vi "Configure Sweep Mode.vi"(5 "Return Time (1s)":dbl[unit]=1.0 format="%#.6g", 7 "Hold Time (0 s)":dbl[unit] format="%#.6g", 8 "error in (no error)":errorcluster, 9 "Sweep Mode (0: Repeated)":u16(ring) items=["Repeated", "Triggered"], 10 "Channel  (0: Channel 1)":T1 items=["Channel 1", "Channel 2"], 11 "VISA resource name":refnum<visa-resource-name>) -> (0 "error out":errorcluster, 3 "VISA resource name out":refnum<visa-resource-name>)   [LabVIEW 2009, in "Tektronix AFG 3000 Series.lvlib"]
doc: "Configures the sweep mode. The VI decides whether the function generator produces a sweep when it receives a trigger or continuous sweep at a rate spedified by sweep time, hold time and return time."
uses:
  Tektronix AFG 3000 Series.lvlib
  controls.llb/Channel.ctl
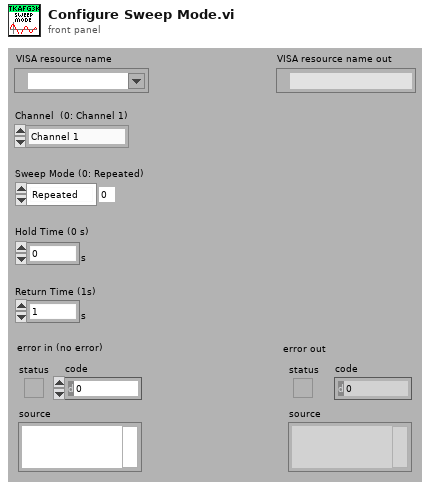
[diagram p1: front panel]
types:
  T1 = typedef "Channel.ctl" = u16
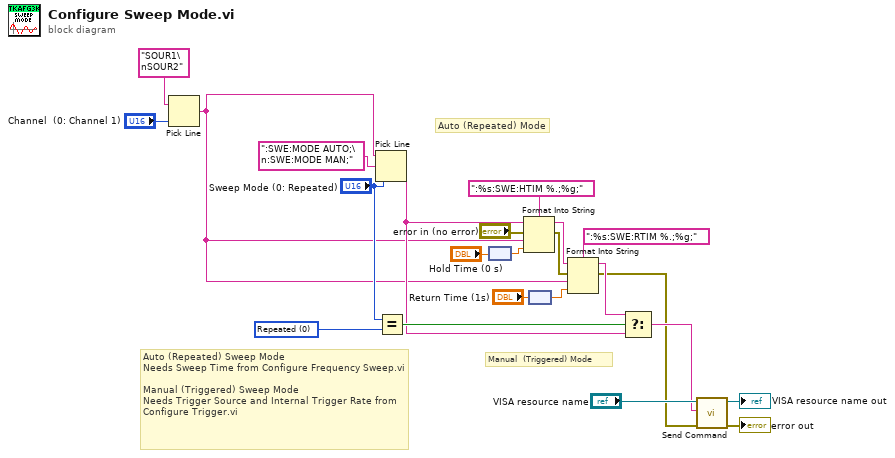
[diagram p0: block diagram]
diagram:
  w22 = u16 0 items=["Repeated", "Triggered"] ("Sweep Mode (0: Repeated)")
  # "Manual  (Triggered) Mode"
  # "Auto (Repeated) Mode"
  # "Auto (Repeated) Sweep Mode\nNeeds Sweep Time from Configure Frequency Sweep.vi\n\nManual (Triggered) Sweep Mode\nNeeds Trigger Source and Internal Trigger Rate from\nConfigure Trigger.vi"
  n1 = Pick Line(multi-line string="SOUR1\nSOUR2" ("string (\"\")"), line index="Channel  (0: Channel 1)") -> (output string=w12:string)  [unwired: 1 out]
  n2 = Pick Line(string ("")=w12, multi-line string=":SWE:MODE AUTO;\n:SWE:MODE MAN;", line index="Sweep Mode (0: Repeated)") -> (output string=w14:string)
  n3 = Equal?(x="Sweep Mode (0: Repeated)", y=w22) -> (x = y?=w19:bool)
  n4 = node("Hold Time (0 s)") -> (w7:dbl)
  n5 = Format Into String(format string=":%s:SWE:HTIM %.;%g;", initial string=w14, error in="error in (no error)", w12, w7) -> (resulting string=w21:string, error out=w10:errorcluster)
  n6 = node("Return Time (1s)") -> (w8:dbl)
  n7 = Format Into String(format string=":%s:SWE:RTIM %.;%g;", initial string=w21, error in=w10, w12, w8) -> (resulting string=w17:string, error out=w1:errorcluster)
  n8 = Select(t=w17, s=w19, f=w14) -> (s? t:f=w2:string)
  n9 = call "Send Command.vi"("error in (no error)"=w1, "write buffer"=w2, "VISA resource name"="VISA resource name") -> ("error out"=→"error out":errorcluster, "VISA resource name out"=→"VISA resource name out":refnum<visa-resource-name>)  [unwired: 7 out]
